vi "Autonomous Independent.vi"() -> ()   [LabVIEW 2017]
doc: "This VI is called when autonomous begins, and will automatically be terminated when autonomous ends. You can carry out timed or sensor driven robot movement independently without needing to return to the caller."
uses:
  Robot Global Data.vi
  <vilib>/Rock Robotics/Network Tables/NT Read String.vi
  LabVIEW_is_Under_Control.lib/Util/Unpack Gamepad/Button Cluster.ctl
panel:
  in  "averege off":bool
  in  "reset encoder":bool
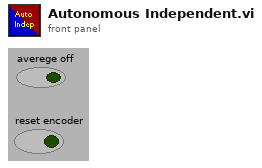
[diagram p1: front panel]
types:
  T1 = typedef "WPI_EncoderDevRef.ctl" = cluster{"DevStatus":errorcluster, "EncoderIndex":T2, "CounterIndex":T3, "DistancePerCount":dbl, "Decoding Type":T4}
  T2 = typedef "FPGA_EncoderIdx.ctl" = enum8{"Enc 0", "Enc 1", "Enc 2", "Enc 3", "Enc 4", "Enc 5", "Enc 6", "Enc 7", "Invalid"}
  T3 = typedef "FPGA_CounterCtrSystemIndex.ctl" = enum8{"Ctr 0", "Ctr 1", "Ctr 2", "Ctr 3", "Ctr 4", "Ctr 5", "Ctr 6", "Ctr 7", "Invalid"}
  T4 = typedef "WPI_EncoderType.ctl" = enum16{"1x", "2x", "4x"}
  T5 = enum16{"AndarFrente", "Parar", "VirarDireita", "AndarFrente2", "LevantarElevador", "Expelir", "Finale"}
  T6 = typedef "Button Cluster.ctl" = cluster{"Buttons[0]":bool, "Buttons[1]":bool, "Buttons[2]":bool, "Buttons[3]":bool, "Buttons[4]":bool, "Buttons[5]":bool, "Buttons[6]":bool, "Buttons[7]":bool, "Buttons[8]":bool, "Buttons[9]":bool}
  T7 = cluster{"proportional gain (Kc)":dbl, "integral time (Ti, min)":dbl, "derivative time (Td, min)":dbl}
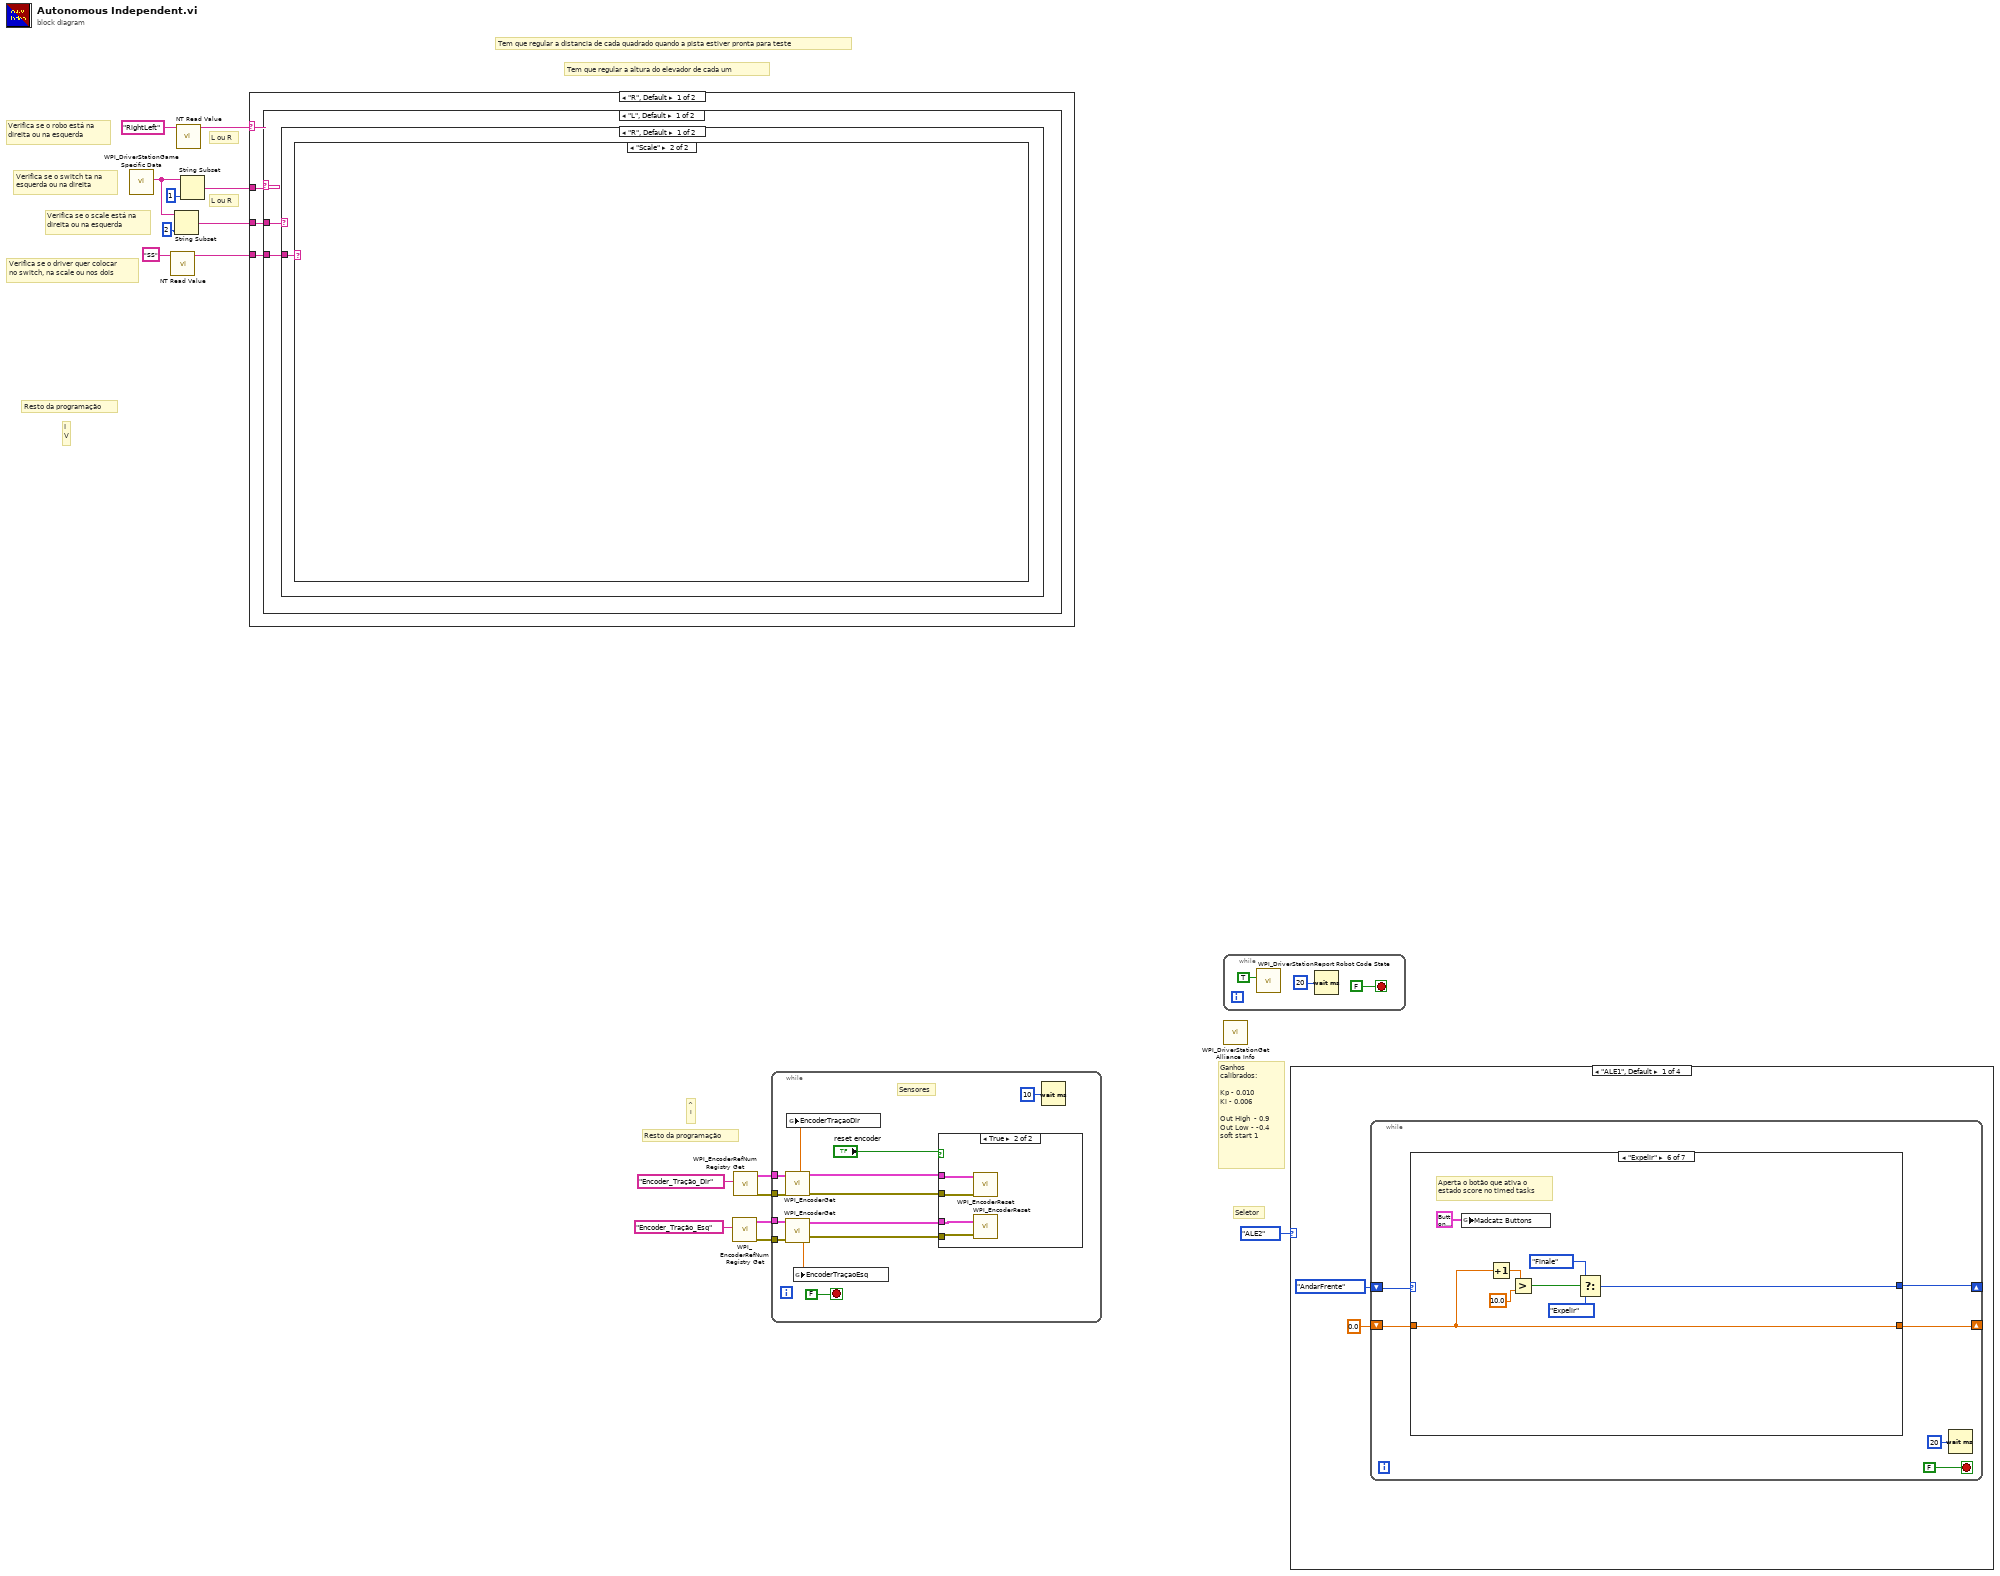
[diagram p0: block diagram]
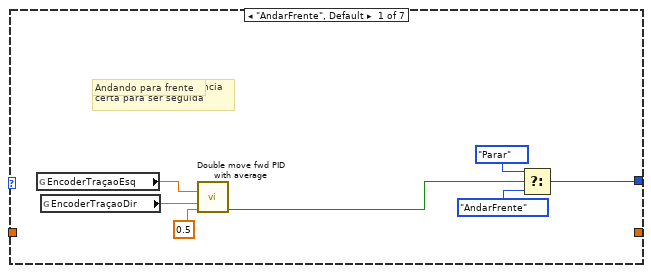
[diagram p19: hidden frame]
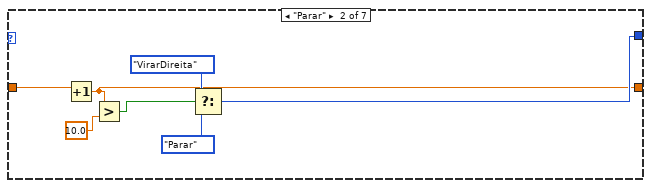
[diagram p20: hidden frame]
diagram:
  # "Tem que regular a altura do elevador de cada um"
  # "Tem que regular a distancia de cada quadrado quando a pista estiver pronta para teste"
  # "Resto da programação"
  # "^\n I"
  # "L ou R"
  # "L ou R"
  # "Resto da programação"
  # "I\nV"
  # "Verifica se o driver quer colocar\nno switch, na scale ou nos dois"
  # "Verifica se o scale está na\ndireita ou na esquerda"
  # "Verifica se o switch ta na\nesquerda ou na direita"
  # "Verifica se o robo está na\ndireita ou na esquerda"
  # "Ganhos calibrados:\n\nKp - 0.010\nKi - 0.006\n\nOut High  - 0.9\nOut Low - -0.4\nsoft start 1"
  # "Seletor"
  n1 = call <vilib>:"WPI_DriverStationGame Specific Data.vi"() -> ("Game Specific Data"=w4:string)  [unwired: 11 in]
  n2 = call-poly <vilib>:"NT Read Value.vi"("Name"="SS") -> ("String"=w1:string)  [unwired: 9 in, 1 out]
  n3 = String Subset(string=w4, length (rest)=2 ("length (rest)")) -> (substring=w3:string)  [unwired: 1 in]
  n4 = call-poly <vilib>:"NT Read Value.vi"("Name"="RightLeft") -> ("String"=w8:string)  [unwired: 9 in, 1 out]
  n5 = String Subset(string=w4, length (rest)=1 ("length (rest)")) -> (substring=w6:string)  [unwired: 1 in]
  n6 = case shown="\"R\", Default" w8 {
    tunnel: w6 -> [w19 w30]
    tunnel: w3 -> [w18 w29]
    tunnel: w1 -> [w17 w28]
    frame "R", Default {
      n7 = case shown="\"L\", Default" w19 {
        tunnel: w18 -> [w21 w25]
        tunnel: w17 -> [w20 w24]
        frame "L", Default {
          n8 = case shown="\"R\", Default" w21 {
            tunnel: w20 -> [w22 w23]
            frame "R", Default {
              n9 = case shown="\"Scale\"" w22 {
                frame "Switch", Default {
                }
                frame "Scale" {
                }
              }
            }
            frame "L" {
              n10 = case shown="\"Scale\", Default" w23 {
                frame "Scale", Default {
                }
                frame "Switch" {
                }
              }
            }
          }
        }
        frame "R" {
          n11 = case shown="\"R\"" w25 {
            tunnel: w24 -> [w26 w27]
            frame "R" {
              n12 = case shown="\"SwitchScale\"" w26 {
                frame "Scale", Default {
                }
                frame "SwitchScale" {
                }
                frame "Switch" {
                }
              }
            }
            frame "L", Default {
              n13 = case shown="\"Switch\"" w27 {
                frame "Scale", Default {
                }
                frame "Switch" {
                }
              }
            }
          }
        }
      }
    }
    frame "L" {
      n14 = case shown="\"R\", Default" w30 {
        tunnel: w29 -> [w32 w36]
        tunnel: w28 -> [w31 w35]
        frame "R", Default {
          n15 = case shown="\"R\", Default" w32 {
            tunnel: w31 -> [w33 w34]
            frame "R", Default {
              n16 = case shown="\"Scale\"" w33 {
                frame "Switch", Default {
                }
                frame "Scale" {
                }
              }
            }
            frame "L" {
              n17 = case shown="\"Switch\", Default" w34 {
                frame "Switch", Default {
                }
                frame "Scale" {
                }
              }
            }
          }
        }
        frame "L" {
          n18 = case shown="\"L\"" w36 {
            tunnel: w35 -> [w37 w38]
            frame "R", Default {
              n19 = case shown="\"Scale\", Default" w37 {
                frame "Scale", Default {
                }
                frame "Switch" {
                }
              }
            }
            frame "L" {
              n20 = case shown="\"SwitchScale\"" w38 {
                frame "Switch", Default {
                }
                frame "Scale" {
                }
                frame "SwitchScale" {
                }
              }
            }
          }
        }
      }
    }
  }
  n21 = call <vilib>:"WPI_EncoderRefNum Registry Get.vi"("refnum name"="Encoder_Tração_Esq") -> ("error out"=w12:errorcluster, "EncoderDevRef"=w11:T1)  [unwired: 9 in]
  n22 = call <vilib>:"WPI_EncoderRefNum Registry Get.vi"("refnum name"="Encoder_Tração_Dir") -> ("error out"=w13:errorcluster, "EncoderDevRef"=w14:T1)  [unwired: 9 in]
  n23 = while {
    tunnel: w14 -> [w51]
    tunnel: w13 -> [w50]
    tunnel: w11 -> [w46]
    tunnel: w12 -> [w47]
    stop <- FALSE stop-if-true
    # "Sensores"
    n24 = call <vilib>:"WPI_EncoderGet.vi"("error in (no error)"=w50, "EncoderDevRef"=w51) -> ("error out"=w42:errorcluster, "Distance"=w49:dbl, "EncoderDevRef"=w43:T1)  [unwired: 4 in, 3 out]
    n25 = call <vilib>:"WPI_EncoderGet.vi"("error in (no error)"=w47, "EncoderDevRef"=w46) -> ("error out"=w40:errorcluster, "Distance"=w48:dbl, "EncoderDevRef"=w41:T1)  [unwired: 4 in, 3 out]
    n26 = global write "Robot Global Data.vi" "EncoderTraçaoDir"(w49) -> ()
    n27 = global write "Robot Global Data.vi" "EncoderTraçaoEsq"(w48) -> ()
    n28 = case shown="True" "reset encoder" {
      tunnel: w43 -> [_ w55]
      tunnel: w42 -> [_ w54]
      tunnel: w41 -> [_ w53]
      tunnel: w40 -> [_ w52]
      frame False {
      }
      frame True {
        n29 = call <vilib>:"WPI_EncoderReset.vi"("error in (no error)"=w54, "EncoderDevRef"=w55) -> ()  [unwired: 8 in, 2 out]
        n30 = call <vilib>:"WPI_EncoderReset.vi"("error in (no error)"=w52, "EncoderDevRef"=w53) -> ()  [unwired: 8 in, 2 out]
      }
    }
    n31 = Wait (ms)(milliseconds to wait=u32 10) -> ()  [unwired: 1 out]
  }
  n32 = call <vilib>:"WPI_DriverStationGet Alliance Info.vi"() -> ()  [unwired: 12 out]
  n33 = while {
    stop <- FALSE stop-if-true
    n34 = call <vilib>:"WPI_DriverStationReport Robot Code State.vi"("Autonomous"=TRUE) -> ()  [unwired: 10 in, 1 out]
    n35 = Wait (ms)(milliseconds to wait=u32 20) -> ()  [unwired: 1 out]
  }
  n36 = case shown="\"ALE1\", Default" enum16{"ALE1", "ALE2", "ALEX", "ALE1X"}."ALE2" {
    frame "ALE1", Default {
      n37 = while {
        shift-right: [w64] -> _
        shift-left: T5."AndarFrente" -> [w65]
        shift-right: [w62] -> _
        shift-left: 0.0 -> [w63]
        stop <- FALSE stop-if-true
        n38 = case shown="\"Expelir\"" w65 {
          tunnel: [w71 w75 w81 w85 _ w91 T5."Finale"] -> w64
          tunnel: w63 -> [_ w80 _ _ _ w92 _]
          tunnel: [_ w74 _ _ _ w92 _] -> w62
          frame "AndarFrente", Default {
            # "Precisa colocar a distancia\ncerta para ser seguida"
            # "Andando para frente"
            n39 = global read "Robot Global Data.vi" "EncoderTraçaoEsq"() -> (w68:dbl)
            n40 = global read "Robot Global Data.vi" "EncoderTraçaoDir"() -> (w67:dbl)
            n41 = call "Double move fwd PID with average.vi"("Encoder Left"=w68, "Encoder Right"=w67, "Precision"=0.5) -> ("finished?"=w69:bool)  [unwired: 11 in, 1 out]
            n42 = Select(t=T5."Parar", s=w69, f=T5."AndarFrente") -> (s? t:f=w71:T5)
          }
          frame "Parar" {
            n43 = Increment(x=w80) -> (x+1=w74:dbl)
            n44 = Greater?(x=w74, y=10.0) -> (0:w79:bool)
            n45 = Select(t=T5."VirarDireita", s=w79, f=T5."Parar") -> (s? t:f=w75:T5)
          }
          frame "VirarDireita" {
            n46 = call "Turn on point PID.vi"() -> ("Finished?"=w84:bool)  [unwired: 9 in, 2 out]
            n47 = Select(t=T5."AndarFrente2", s=w84, f=T5."VirarDireita") -> (s? t:f=w81:T5)
          }
          frame "AndarFrente2" {
            # "Precisa colocar a distancia certa"
            n48 = global read "Robot Global Data.vi" "EncoderTraçaoEsq"() -> (w90:dbl)
            n49 = global read "Robot Global Data.vi" "EncoderTraçaoDir"() -> (w89:dbl)
            n50 = call "Double move fwd PID with average.vi"("Encoder Left"=w90, "Encoder Right"=w89) -> ("finished?"=w88:bool)  [unwired: 12 in, 1 out]
            n51 = Select(t=T5."LevantarElevador", s=w88, f=T5."AndarFrente2") -> (s? t:f=w85:T5)
          }
          frame "LevantarElevador" {
            # "Levantar o elevador\n\n//A programação do\nelevador ainda n foi feita"
          }
          frame "Expelir" {
            # "Aperta o botão que ativa o\nestado score no timed tasks"
            n52 = global write "Robot Global Data.vi" "Madcatz Buttons"(T6 {"Buttons[0]"=FALSE, "Buttons[1]"=FALSE, "Buttons[2]"=FALSE, "Buttons[3]"=FALSE, "Buttons[4]"=TRUE, "Buttons[5]"=FALSE, "Buttons[6]"=FALSE, "Buttons[7]"=FALSE, "Buttons[8]"=FALSE, "Buttons[9]"=FALSE} ("Madcatz Buttons")) -> ()
            n53 = Increment(x=w92) -> (x+1=w93:dbl)
            n54 = Greater?(x=w93, y=10.0) -> (0:w97:bool)
            n55 = Select(t=T5."Finale", s=w97, f=T5."Expelir") -> (s? t:f=w91:T5)
          }
          frame "Finale" {
          }
        }
        n56 = Wait (ms)(milliseconds to wait=u32 20) -> ()  [unwired: 1 out]
      }
    }
    frame "ALE2" {
      n57 = case shown="False" "averege off" {
        frame False {
          n58 = while {
            stop <- FALSE stop-if-true
            w105 = u32 10 ("milliseconds to wait")
            n59 = global read "Robot Global Data.vi" "EncoderTraçaoEsq"() -> (w107:dbl)
            n60 = global read "Robot Global Data.vi" "EncoderTraçaoDir"() -> (w108:dbl)
            n61 = Wait (ms)(milliseconds to wait=w105) -> ()  [unwired: 1 out]
            n62 = call "Double move fwd PID with average.vi"("Distance"=300.0, "Gains"=T7 {"proportional gain (Kc)"=0.01, "integral time (Ti, min)"=0.006, "derivative time (Td, min)"=0.0}, "Range"=cluster{"output high":dbl, "output low":dbl} {"output high"=0.9, "output low"=-0.4}, "Encoder Left"=w107, "Encoder Right"=w108, "Precision"=0.5, "Loop Timer"=w105, "Time to stop"=1000) -> ("PWM out"=w101:dbl)  [unwired: 6 in, 1 out]
            n63 = global write "Robot Global Data.vi" "Left Tração Value"(w101) -> ()
            n64 = global write "Robot Global Data.vi" "Right Tração Value"(w101) -> ()
          }
        }
        frame True {
          n65 = while {
            stop <- FALSE stop-if-true
            w116 = u32 10 ("milliseconds to wait")
            n66 = global read "Robot Global Data.vi" "EncoderTraçaoEsq"() -> (w118:dbl)
            n67 = global read "Robot Global Data.vi" "EncoderTraçaoDir"() -> (w119:dbl)
            n68 = Wait (ms)(milliseconds to wait=w116) -> ()  [unwired: 1 out]
            n69 = call "Double move fwd PID.vi"("Time to stop"=1000, "Range"=cluster{"output high":dbl, "output low":dbl} {"output high"=0.9, "output low"=-0.4}, "Loop Timer"=w116, "Gains"=T7 {"proportional gain (Kc)"=0.01, "integral time (Ti, min)"=0.006, "derivative time (Td, min)"=0.0}, "Precision"=0.5, "Encoder Right"=w119, "Encoder Left"=w118, "Distance"=300.0) -> ("PWM Right"=w111:dbl, "PWM Left"=w112:dbl)  [unwired: 1 in, 1 out]
            n70 = global write "Robot Global Data.vi" "Left Tração Value"(w112) -> ()
            n71 = global write "Robot Global Data.vi" "Right Tração Value"(w111) -> ()
          }
        }
      }
    }
    frame "ALEX" {
    }
    frame "ALE1X" {
    }
  }
